vi "spin_flip.vi"() -> ()   [LabVIEW 2012]
uses:
  <vilib>/DAQmx/create/channels.llb/DAQmx Create Channel (CO-Pulse Generation-Frequency).vi
  <vilib>/DAQmx/configure/timing.llb/DAQmx Timing (Implicit).vi
  <vilib>/Utility/file.llb/Write To Spreadsheet File (DBL).vi
  <vilib>/Analysis/NI_AALBase.lvlib
panel:
  out "Dark Counts":i32
  out "Bright Counts":u32=198
  out "XY Graph":cluster{"Y":dbl[], "Y":dbl[]}[](graph)
  out "Frequency":dbl format="%#_6f"
  in  "Frequency Step":dbl
  in  "Stop Frequency":dbl format="%#_6f"
  in  "Start Frequency":dbl format="%#_6f"
  in  "Save data to":path
  out "Fluorescence Before":T1(graph)
  in  "Fluoresence Threshold":u32
  out "Fluorescence After":T1(graph)
  in  "Runs":i32
  in  "stop":bool
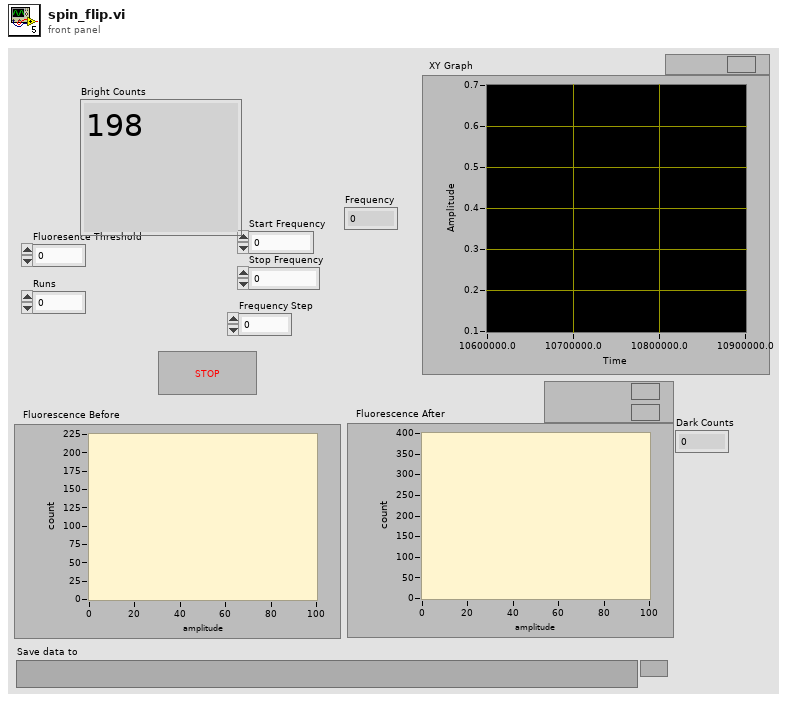
[diagram p1: front panel]
types:
  T1 = cluster{"X Values":dbl[], "Histogram: h(x)":i32[]}
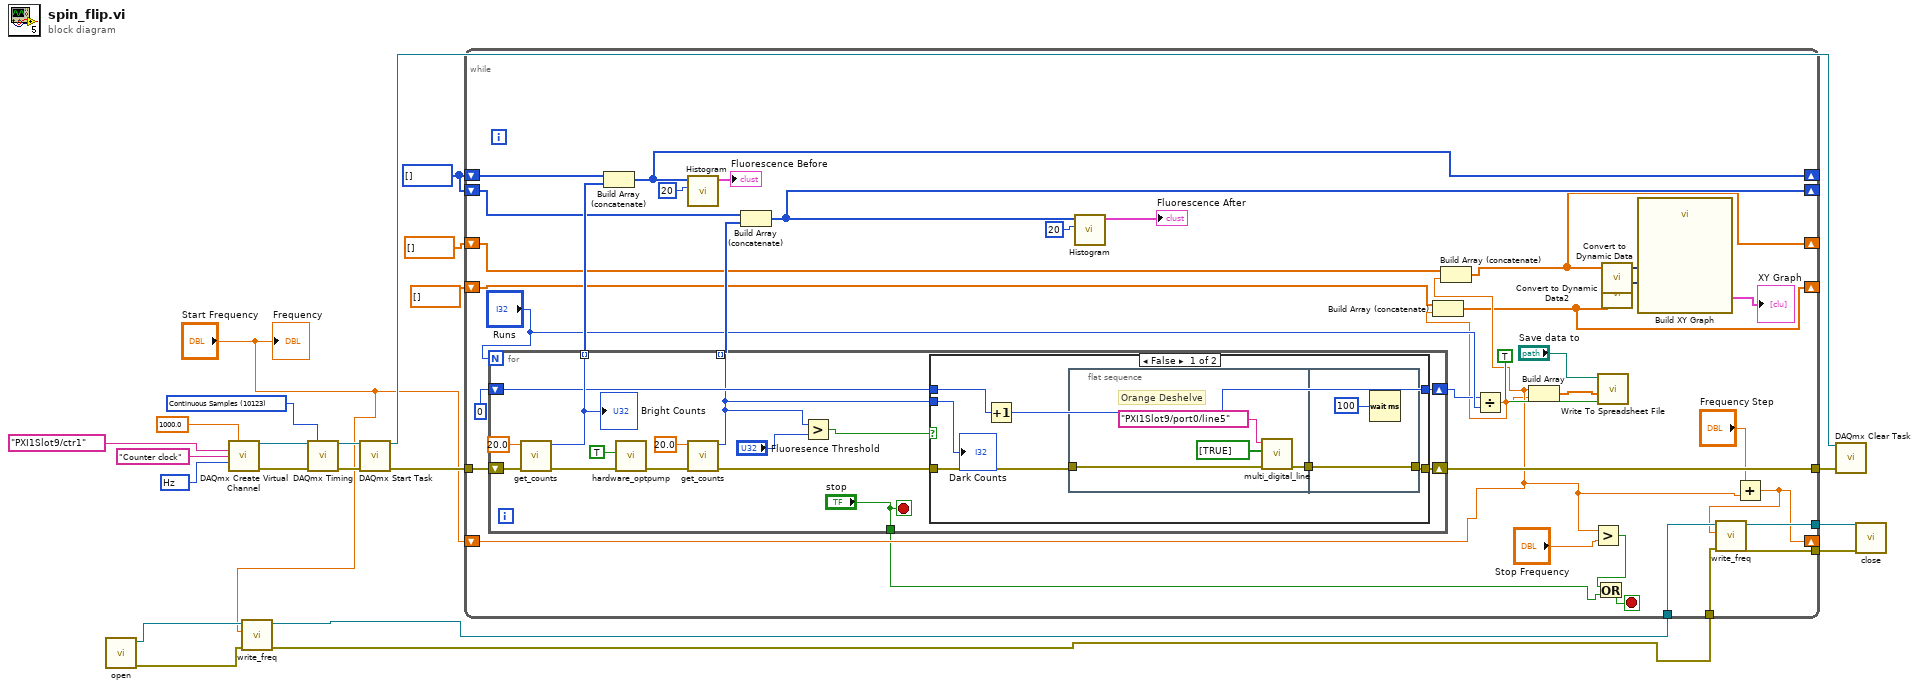
[diagram p0: block diagram]
diagram:
  w11 = i32[] [] ("initialized array")
  w17 = 10123 items=["Finite Samples"=10178, "Continuous Samples"=10123, "Hardware Timed Single Point"=12522] ("sample mode")
  w22 = 10373 items=["Hz"=10373] ("units")
  n1 = call "open.vi"() -> ("error out"=w6:errorcluster, "VISA resource name out"=w7:refnum<visa-resource-name>)  [unwired: 9 in, 1 out]
  n2 = call-poly <vilib>:"DAQmx Create Virtual Channel.vi"("frequency"=1000.0 ("rate"), "counter"=tag "PXI1Slot9/ctr1", "name to assign"="Counter clock", "units"=w22) -> ("task out"=w21:refnum<k21>, "error out"=w20:errorcluster)  [unwired: 10 in]
  n3 = call "write_freq.vi"("error in (no error)"=w6, "number"="Start Frequency", "VISA Refnum in"=w7) -> ("error out"=w4:errorcluster, "VISA Refnum out"=w3:refnum<visa-resource-name>)  [unwired: 7 in]
  n4 = call-poly <vilib>:"DAQmx Timing.vi"("task/channels in"=w21, "sample mode"=w17, "error in"=w20) -> ("task out"=w19:refnum<k21>, "error out"=w18:errorcluster)  [unwired: 11 in]
  n5 = call <vilib>:"DAQmx Start Task.vi"("task/channels in"=w19, "error in"=w18) -> ("task out"=w12:refnum<k21>, "error out"=w13:errorcluster)  [unwired: 12 in]
  n6 = while {
    tunnel: w13 -> [w44]
    tunnel: [w59] -> w10
    shift-right: [w47] -> _
    shift-left: w11 -> [w50]
    shift-right: [w51] -> _
    shift-left: w11 -> [w52]
    tunnel: w3 -> [w40]
    tunnel: w4 -> [w39]
    tunnel: [w38] -> w9
    tunnel: [w37] -> w8
    shift-right: [w34] -> _
    shift-left: "Start Frequency" -> [w29]
    shift-right: [w24] -> _
    shift-left: dbl[] [] -> [w30]
    shift-right: [w25] -> _
    shift-left: dbl[] [] -> [w31]
    stop <- w45 stop-if-true
    n7 = for {
      N: "Runs" -> [_]
      tunnel: [w68] -> w55 mode=indexing
      tunnel: [w60] -> w49 mode=indexing
      shift-right: [w71] -> w59
      shift-left: w44 -> [w66]
      shift-right: [w62] -> w41
      shift-left: 0 -> [w63]
      tunnel: ["stop"] -> w23
      stop <- "stop" stop-if-true
      n8 = call "get_counts.vi"("error in"=w66, "Detection length (ms)"=20.0) -> ("error out"=w70:errorcluster, "Counts"=w68:u32)  [unwired: 8 in]
      "Bright Counts" <- w68
      n9 = call "hardware_optpump.vi"("error in"=w70, "Pump?"=TRUE) -> ("error out"=w69:errorcluster)  [unwired: 9 in]
      n10 = call "get_counts.vi"("error in"=w69, "Detection length (ms)"=20.0) -> ("error out"=w72:errorcluster, "Counts"=w60:u32)  [unwired: 8 in]
      n11 = Greater?(x=w60, y="Fluoresence Threshold") -> (0:w64:bool)
      n12 = case shown="False" w64 {
        tunnel: w72 -> [w79 w87]
        tunnel: [w78 w87] -> w71
        tunnel: w63 -> [w77 w88]
        tunnel: [w76 w88] -> w62
        tunnel: w60 -> [w75 _]
        frame False {
          n13 = Increment(x=w77) -> (x+1=w76:i32)
          n14 = flat-sequence {
            tunnel: w79 -> [w84]
            tunnel: [w81] -> w80
            tunnel: [w86] -> w78
            tunnel: w80 -> [w86]
            frame #0 {
              # "Orange Deshelve"
              n15 = call "multi_digital_line.vi"("error in"=w84, "data"=bool[] [TRUE], "lines"=tag "PXI1Slot9/port0/line5" ("lines 2")) -> ("error out"=w81:errorcluster)  [unwired: 8 in]
            }
            frame #1 {
              n16 = Wait (ms)(milliseconds to wait=u32 100 ("455 Pumping Time 2")) -> ()  [unwired: 1 out]
            }
          }
          "Dark Counts" <- w75
        }
        frame True {
        }
      }
    }
    n17 = Build Array (concatenate)(w52, w55) -> (w51:u32[])
    n18 = call <vilib>:"Histogram.vi"("intervals"=20, "X"=w51) -> ("Histogram Graph"=→"Fluorescence Before":T1)  [unwired: 6 in, 3 out]
    n19 = Build Array (concatenate)(w50, w49) -> (w47:u32[])
    n20 = call <vilib>:"Histogram.vi"("intervals"=20, "X"=w47) -> ("Histogram Graph"=→"Fluorescence After":T1)  [unwired: 6 in, 3 out]
    n21 = Build Array (concatenate)(w31, w29) -> (w25:dbl[])
    n22 = Divide(x=w41, y="Runs") -> (x/y=w28:dbl)
    n23 = Build Array (concatenate)(w30, w28) -> (w24:dbl[])
    n24 = Build Array(w29, w28) -> (w33:dbl[])
    n25 = Greater?(x=w29, y="Stop Frequency") -> (0:w46:bool)
    n26 = Or(x=w46, y=w23) -> (x .or. y?=w45:bool)
    n27 = call-poly <vilib>:"Write To Spreadsheet File.vi"("append to file? (new file:F)"=TRUE, "1D data"=w33, "file path (dialog if empty)"="Save data to") -> ()  [unwired: 5 in, 1 out]
    n28 = call "Convert to Dynamic Data"("Array"=w25) -> ("Dynamic Data Type"=w27:dynamicdata)  [unwired: 3 in]
    n29 = call "Convert to Dynamic Data2"("Array"=w24) -> ("Dynamic Data Type"=w26:dynamicdata)  [unwired: 3 in]
    n30 = call "Build XY Graph"("Y Input"=w26, "X Input"=w27) -> ("XY Graph"=→"XY Graph":cluster{"Y":dbl[], "Y":dbl[]}[])  [unwired: 3 in, 6 out]
    n31 = Add(x="Frequency Step", y=w29) -> (x+y=w34:dbl)
    n32 = call "write_freq.vi"("error in (no error)"=w39, "number"=w34, "VISA Refnum in"=w40) -> ("error out"=w37:errorcluster, "VISA Refnum out"=w38:refnum<visa-resource-name>)  [unwired: 7 in]
  }
  n33 = call <vilib>:"DAQmx Clear Task.vi"("task in"=w12, "error in"=w10) -> ()  [unwired: 13 in, 1 out]
  n34 = call "close.vi"("error in (no error)"=w8, "VISA resource name"=w9) -> ()  [unwired: 9 in, 1 out]
  "Frequency" <- "Start Frequency"
